vi "UpdataModel.vi"(5 "更新零件信息":T1, 6 "ModelEditInfo in":T2) -> (2 "ModelEditInfo out":T2)   [LabVIEW 2014]
uses:
  <vilib>/Utility/file.llb/Write To Spreadsheet File (string).vi
  ModeEditeControl.ctl
  ModelInfo.ctl
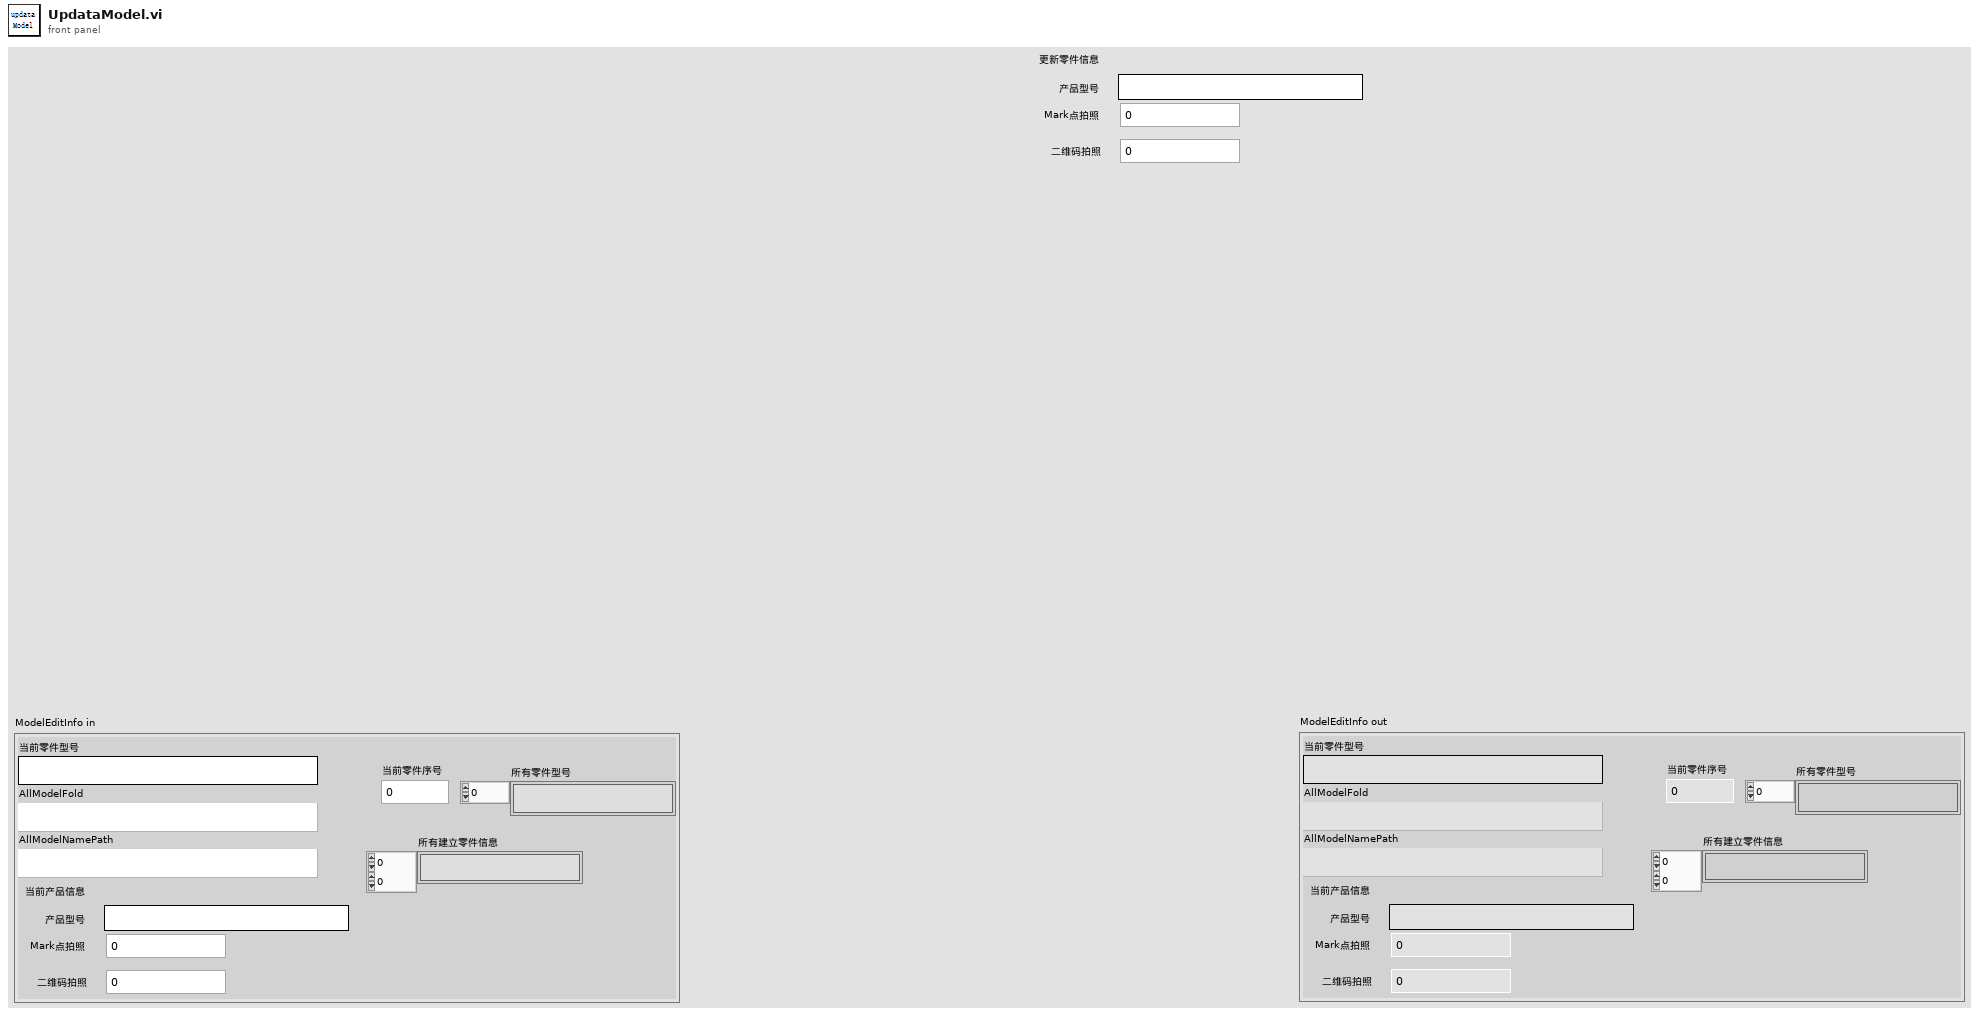
[diagram p1: front panel]
types:
  T1 = typedef "ModelInfo.ctl" = cluster{"产品型号":string, "二维码拍照":u32, "Mark点拍照":u32}
  T2 = typedef "ModeEditeControl.ctl" = cluster{"AllModelFold":path, "AllModelNamePath":path, "所有零件型号":string[], "当前零件型号":string, "所有建立零件信息":string[][], "当前零件序号":i32, "当前产品信息":T1}
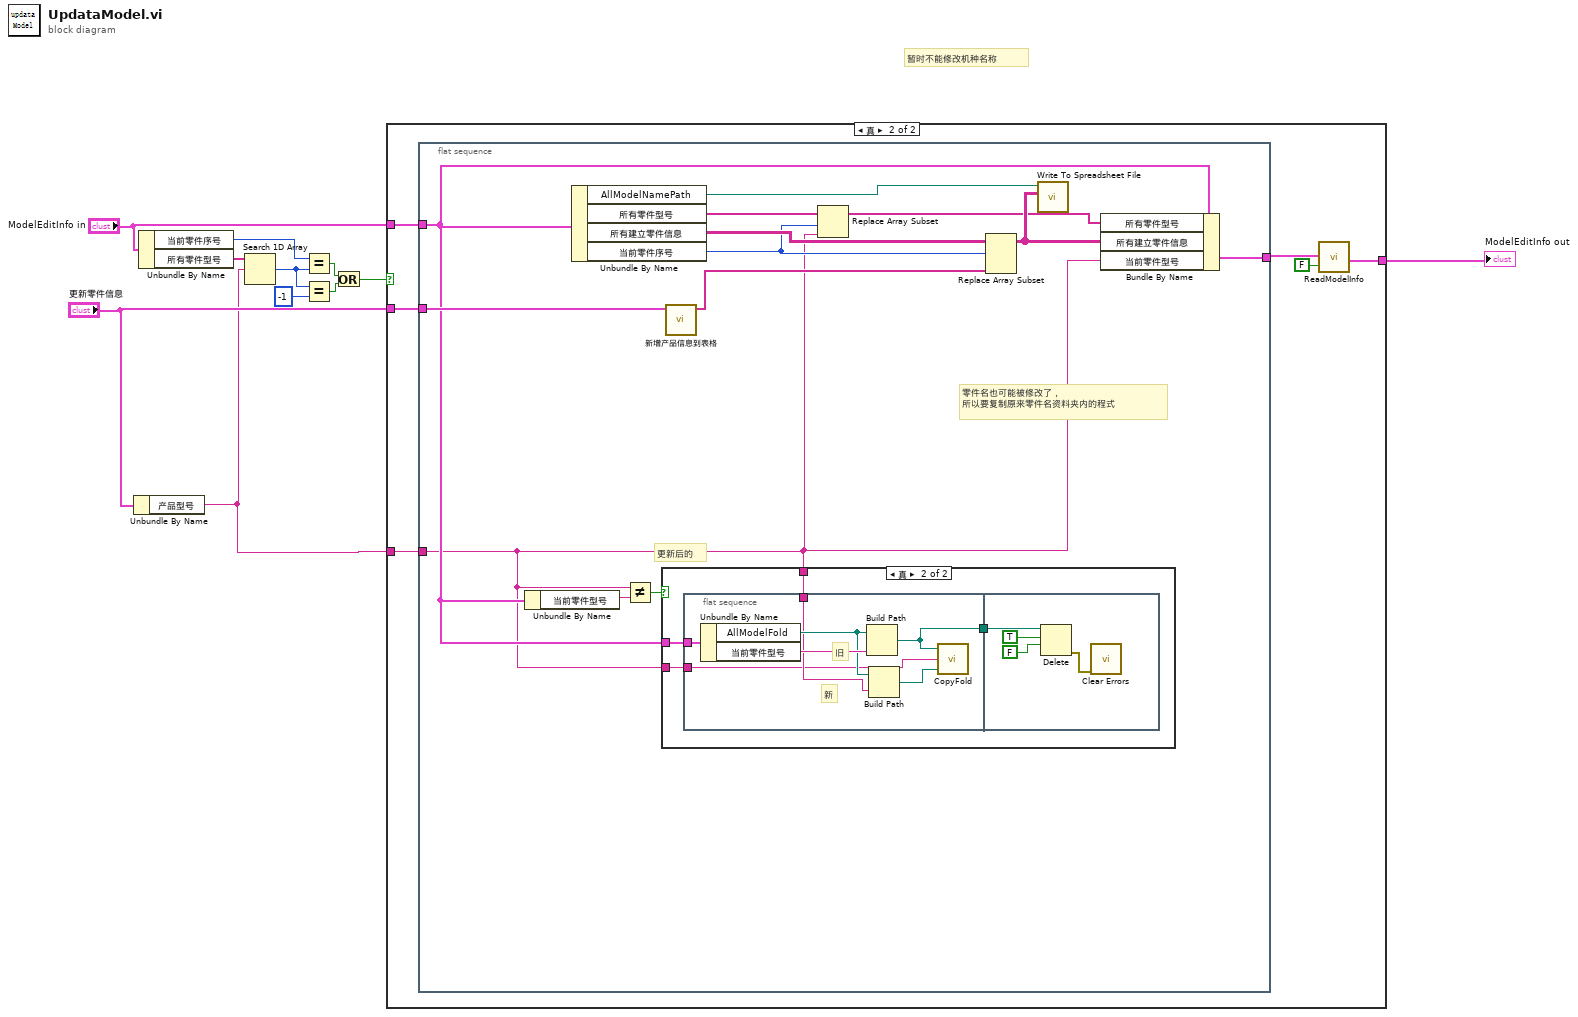
[diagram p0: block diagram]
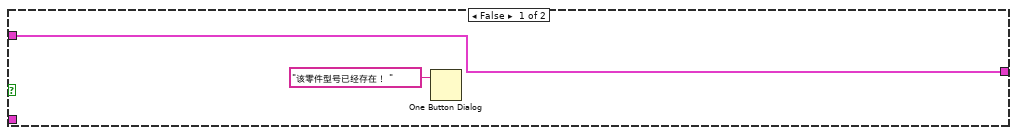
[diagram p2: hidden frame]
diagram:
  # "暂时不能修改机种名称"
  n1 = Unbundle By Name("更新零件信息") -> ("产品型号"=w1:string)
  n2 = Unbundle By Name("ModelEditInfo in") -> ("当前零件序号"=w8:i32, "所有零件型号"=w9:string[])
  n3 = Search 1D Array(1D array=w9, element=w1) -> (index of element=w7:i32)  [unwired: 1 in]
  n4 = Equal?(x=w8, y=w7) -> (x = y?=w5:bool)
  n5 = Equal?(x=w7, y=-1) -> (x = y?=w4:bool)
  n6 = Or(x=w5, y=w4) -> (x .or. y?=w2:bool)
  n7 = case shown="真" w2 {
    tunnel: "更新零件信息" -> [_ w19]
    tunnel: "ModelEditInfo in" -> [w12 w17]
    tunnel: w1 -> [_ w16]
    tunnel: [w12 w15] -> w3
    frame False {
      n8 = One Button Dialog(message="该零件型号已经存在！ " ("消息")) -> ()  [unwired: 1 in, 1 out]
    }
    frame True {
      n9 = flat-sequence {
        tunnel: [w32] -> w18
        tunnel: w17 -> [w21]
        tunnel: w16 -> [w20]
        tunnel: w19 -> [w23]
        frame #0 {
          # "零件名也可能被修改了，\n所以要复制原来零件名资料夹内的程式"
          # "更新后的"
          n10 = Unbundle By Name(w21) -> ("当前零件型号"=w26:string)
          n11 = Unbundle By Name(w21) -> ("AllModelNamePath"=w31:path, "所有零件型号"=w30:string[], "所有建立零件信息"=w29:string[][], "当前零件序号"=w24:i32)
          n12 = Not Equal?(x=w20, y=w26) -> (x != y?=w25:bool)
          n13 = case shown="真" w25 {
            tunnel: w21 -> [_ w36]
            tunnel: w20 -> [_ w35]
            tunnel: w20 -> [_ w34]
            frame False {
              # "零件名称没有变更"
            }
            frame True {
              n14 = flat-sequence {
                tunnel: w36 -> [w43]
                tunnel: w35 -> [w40]
                tunnel: [w38] -> w33
                tunnel: w34 -> [w37]
                tunnel: w33 -> [w47]
                frame #0 {
                  # "新"
                  # "旧"
                  n15 = Unbundle By Name(w43) -> ("AllModelFold"=w41:path, "当前零件型号"=w42:string)
                  n16 = Build Path(base path=w41, name or relative path=w42) -> (appended path=w38:path)
                  n17 = Build Path(base path=w41, name or relative path=w40) -> (appended path=w39:path)
                  n18 = call "CopyFold.vi"("New path"=w39, "新零件型号"=w37, "源 path"=w38) -> ()
                }
                frame #1 {
                  n19 = Delete(path (use dialog)=w47, entire hierarchy (F)=TRUE ("整个层次结构(F)"), confirm (F)=FALSE ("确认(F)")) -> (error out=w44:errorcluster)  [unwired: 2 in, 2 out]
                  n20 = call <vilib>:"Clear Errors.vi"("error in (no error)"=w44) -> ()  [unwired: 5 in, 2 out]
                }
              }
            }
          }
          n21 = call "新增产品信息到表格.vi"("新增零件信息"=w23) -> ("数组"=w22:string[])  [unwired: 10 in]
          n22 = Replace Array Subset(array=w30, new element=w20, index=w24) -> (w27:string[])
          n23 = Replace Array Subset(array=w29, new element=w22, index (row)=w24) -> (w28:string[][])  [unwired: 1 in]
          n24 = call-poly <vilib>:"Write To Spreadsheet File.vi"("2D data"=w28, "file path (dialog if empty)"=w31) -> ()  [unwired: 6 in, 1 out]
          n25 = Bundle By Name(cluster=w21, "所有零件型号"=w27, "所有建立零件信息"=w28, "当前零件型号"=w20) -> (w32:T2)
        }
      }
      n26 = call "ReadModelInfo.vi"("更新量测项目序号"=FALSE, "ModelEditInfo in"=w18) -> ("ModelEditInfo out"=w15:T2)  [unwired: 1 in]
    }
  }
  "ModelEditInfo out" <- w3
